vi "Compute sample count for frequency.vi"(0 "F (sampler)":dbl=3200000000.0 format="%#_13p", 2 "Sample Quantum":i32=32, 5 "desired wfm frequency":dbl format="%#_15p") -> (4 "F (sampler) out":dbl=3200000000.0 format="%#_13p", 6 "least common num samples":i64)   [LabVIEW 2018, in "GettingStarted_5785_Host.lvlib"]
uses:
  GettingStarted_5785_Host.lvlib
  <vilib>/gmath/NI_Gmath.lvlib
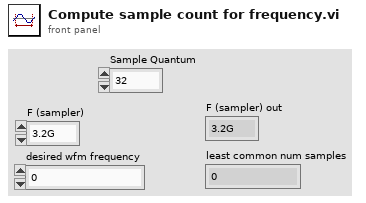
[diagram p1: front panel]
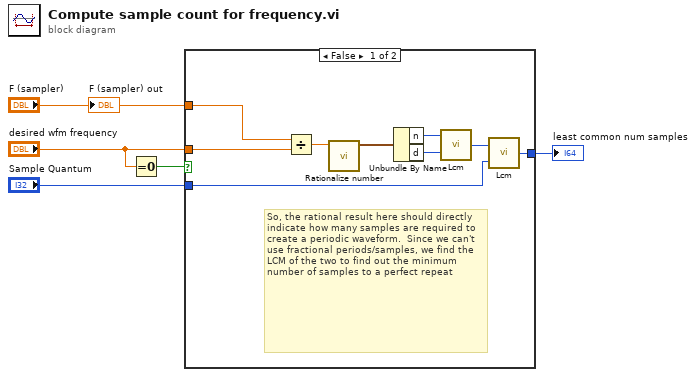
[diagram p0: block diagram]
diagram:
  n1 = Equal To 0?(x="desired wfm frequency") -> (x = 0?=w3:bool)
  n2 = case shown="False" w3 {
    tunnel: "desired wfm frequency" -> [w13 _]
    tunnel: "Sample Quantum" -> [w8 w15]
    tunnel: [w7 w15] -> w4
    tunnel: "F (sampler)" -> [w6 _]
    frame False {
      # "So, the rational result here should directly indicate how many samples are required to create a periodic waveform.  Since we can't use fractional periods/samples, we find the LCM of the two to find out the minimum number of samples to a perfect repeat"
      n3 = Divide(x=w6, y=w13) -> (x/y=w14:dbl)
      n4 = call "Rationalize number.vi"("number in"=w14) -> ("rationalized"=w12:cluster{"n":u64, "d":u64})  [unwired: 10 in]
      n5 = Unbundle By Name(w12) -> ("n"=w11:u64, "d"=w10:u64)
      n6 = call <vilib>:"Lcm.vi"("y"=w10, "x"=w11) -> ("lcm(x,y)"=w9:i64)
      n7 = call <vilib>:"Lcm.vi"("y"=w8, "x"=w9) -> ("lcm(x,y)"=w7:i64)
    }
    frame True {
      # "Allow generating a DC waveform, just use\nthe sample quantum since we won't find\na common multiple with no frequency"
    }
  }
  "least common num samples" <- w4
  "F (sampler) out" <- "F (sampler)"
